vi "DUC (Two Channels).vi"(0 "data":u32[](array[numeric]), 1 "reset":bool, 5 "enable":bool[](array[boolean]), 9 "input valid":bool, 11 "duc parameters":T1[](array[typedef]) {"frequency shift" format="%#.48g"}) -> (4 "I data out":i16[](array[numeric]), 6 "Q data out":i16[](array[numeric]), 13 "dsp reset done":bool, 14 "ready for input":bool, 15 "number of overflows":u64[](array[numeric]))   [LabVIEW 2020]
doc: "Digital upconverter (DUC). Implemented with FPGA-based DSP.\n\n<B>Input Parameters</B>\n\n<B>data in</B> is the I and Q data to be upconverted along with overflow information.\n\n<B>enable</B> specifies which streams are enabled.\n\n<B>input valid</B> specifies when 'data in' is valid.\n\n<B>duc parameters</B> are the upconversion parameters utilized by the DSP chain.\n\n<B>reset</B> the DSP upconversion signal chain.\n\n<B>Output Parameters</B>\n\n<B>dsp reset done</B> indicates that the DSP upconversion signal chain completed reset.\n\n<B>ready for input</B> is a flow control signal that indicates whether the DUC is ready to accept new data.\n\n<B>I data out</B> is the in phase component of upconverted data to be transmitted.\n\n<B>Q data out</B> is the quadrature phase component of upconverted data to be transmitted.\n\n<B>output valid</B> specifies when 'data out' is valid.\n\n<B>number of overflows</B> is the number of times the DSP chain overflowed on fixed point conversion of 'data in'."
uses:
  DUC Parameters.ctl
  <instrlib>/_niInstr/DSP/v1/Shared/Public/IQ Impairments.ctl
  <instrlib>/_niInstr/DSP/v1/Shared/Public/IQ Gain.ctl
  <instrlib>/_niInstr/DSP/v1/Shared/niInstr DSP v1 Shared.lvlib
panel:
  out "output valid":bool
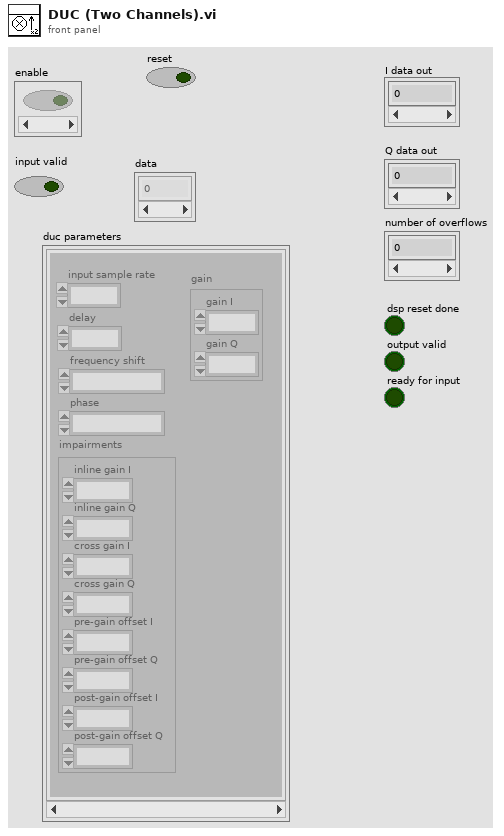
[diagram p1: front panel]
types:
  T1 = typedef "DUC Parameters.ctl" = cluster{"frequency shift":fxp<+/-,48,0>, "impairments":T2, "phase":fxp<+/-,21,0>, "input sample rate":fxp<+,48,1>, "gain":T3, "delay":fxp<+/-,18,0>}
  T2 = typedef "niInstr DSP v1 Shared.lvlib/IQ Impairments.ctl" = cluster{"inline gain I":fxp<+/-,18,1>, "inline gain Q":fxp<+/-,18,1>, "cross gain I":fxp<+/-,18,1>, "cross gain Q":fxp<+/-,18,1>, "pre-gain offset I":fxp<+/-,18,1>, "pre-gain offset Q":fxp<+/-,18,1>, "post-gain offset I":fxp<+/-,18,1>, "post-gain offset Q":fxp<+/-,18,1>}
  T3 = typedef "niInstr DSP v1 Shared.lvlib/IQ Gain.ctl" = cluster{"gain I":fxp<+/-,24,3>, "gain Q":fxp<+/-,24,3>}
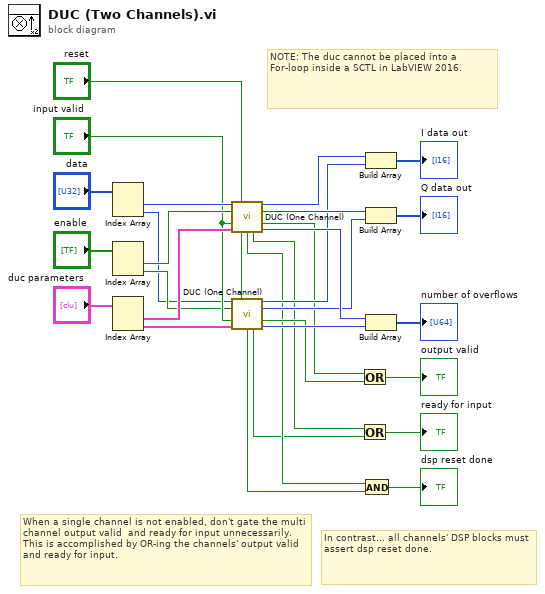
[diagram p0: block diagram]
diagram:
  # "NOTE: The duc cannot be placed into a For-loop inside a SCTL in LabVIEW 2016."
  # "When a single channel is not enabled, don't gate the multi channel output valid  and ready for input unnecessarily.  This is accomplished by OR-ing the channels' output valid and ready for input."
  # "In contrast... all channels' DSP blocks must assert dsp reset done."
  n1 = Index Array(array="data") -> (element #1=w24:u32, element #2=w16:u32)  [unwired: 2 in]
  n2 = Index Array(array="enable") -> (element #1=w23:bool, element #2=w17:bool)  [unwired: 2 in]
  n3 = Index Array(array="duc parameters") -> (element #1=w20:T1, element #2=w19:T1)  [unwired: 2 in]
  n4 = call "DUC (One Channel).vi"("data"=w24, "reset"="reset", "enable"=w23, "input valid"="input valid", "duc parameters"=w20) -> ("I data out"=w15:i16, "Q data out"=w11:i16, "output valid"=w6:bool, "dsp reset done"=w3:bool, "ready for input"=w4:bool, "number of overflows"=w12:u64)  [unwired: 5 in]
  n5 = call "DUC (One Channel).vi"("data"=w16, "reset"="reset", "enable"=w17, "input valid"="input valid", "duc parameters"=w19) -> ("I data out"=w9:i16, "Q data out"=w10:i16, "output valid"=w5:bool, "dsp reset done"=w1:bool, "ready for input"=w2:bool, "number of overflows"=w14:u64)  [unwired: 5 in]
  n6 = Or(x=w6, y=w5) -> (x .or. y?=→"output valid":bool)
  n7 = Or(x=w4, y=w2) -> (x .or. y?=→"ready for input":bool)
  n8 = And(x=w3, y=w1) -> (x .and. y?=→"dsp reset done":bool)
  n9 = Build Array(w15, w9) -> (→"I data out":i16[])
  n10 = Build Array(w11, w10) -> (→"Q data out":i16[])
  n11 = Build Array(w12, w14) -> (→"number of overflows":u64[])
